vi "Parse Text.vi"(8 "Error In":errorcluster) -> (0 "Error Out":errorcluster)   [LabVIEW 2017, in "Tests.lvlib"]
uses:
  Tests.lvlib
  src/Mustache/Public/Readers/Public/String/String.lvclass
  D:/Users/cfield/Code/Field R&D Services/Mustache/feature-lv-original-parser/src/Mustache/Public/Readers/Public/Abstract/Abstract.lvclass
  <vilib>/addons/_JKI Toolkits/Caraya/classes/Test/Test.lvclass
  src/Mustache/Public/Parser/Parser.lvclass
  <vilib>/addons/_JKI Toolkits/Caraya/classes/Assert/Assert.lvclass
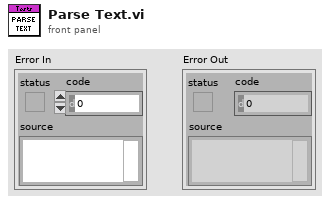
[diagram p1: front panel]
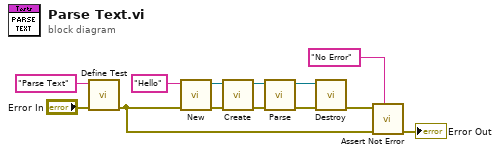
[diagram p0: block diagram]
diagram:
  n1 = call <vilib>:"Define Test.vi"("error in (no error)"="Error In", "Label (VI Title)"="Parse Text") -> ("error out"=w3:errorcluster)  [unwired: 9 in]
  n2 = call "New.vi"("Error In"=w3, "String"="Hello") -> ("Error Out"=w9:errorcluster, "String"=w10:refnum<class "String.lvclass">)  [unwired: 8 in]
  n3 = call "Create.vi"("Error In"=w9, "Reader"=w10) -> ("Error Out"=w8:errorcluster, "Parser"=w7:refnum<class "Parser.lvclass">)  [unwired: 8 in]
  n4 = call "Parse.vi"("Error In"=w8, "Parser In"=w7) -> ("Error Out"=w5:errorcluster, "Parser Out"=w6:refnum<class "Parser.lvclass">)  [unwired: 7 in, 1 out]
  n5 = call "Destroy.vi"("Error In"=w5, "Parser"=w6) -> ("Error Out"=w4:errorcluster)  [unwired: 9 in]
  n6 = call <vilib>:"Assert Not Error.vi"("Label"="No Error", "error in (no error)"=w3, "Not Error?"=w4) -> ("error out"=→"Error Out":errorcluster)  [unwired: 8 in]
